vi "Main.vi"() -> ()   [LabVIEW 2019]
uses:
  Controls/State.ctl
  <vilib>/MediaMongrels Ltd/WebSockets/WebSockets/WebSocket Server/WebSocket Server.lvclass
  <vilib>/MediaMongrels Ltd/WebSockets/Sockets/VISA TCP Listener/VISA TCP Listener.lvclass
panel:
  in  "Stop":bool
  out "Current Time":string
  # "Raspberry Pi WebSocket Server Example"
  # "This simple example sends the current date/time to the connected WebSocket Client.\n\nTo be used in conjunction with the corresponding NXG WebVI."
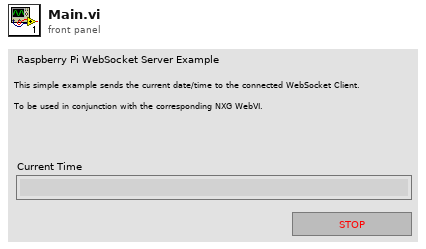
[diagram p1: front panel]
types:
  T1 = typedef "State.ctl" = enum16{"Initialise", "Listen", "Write Data", "Close WebSocket", "Exit"}
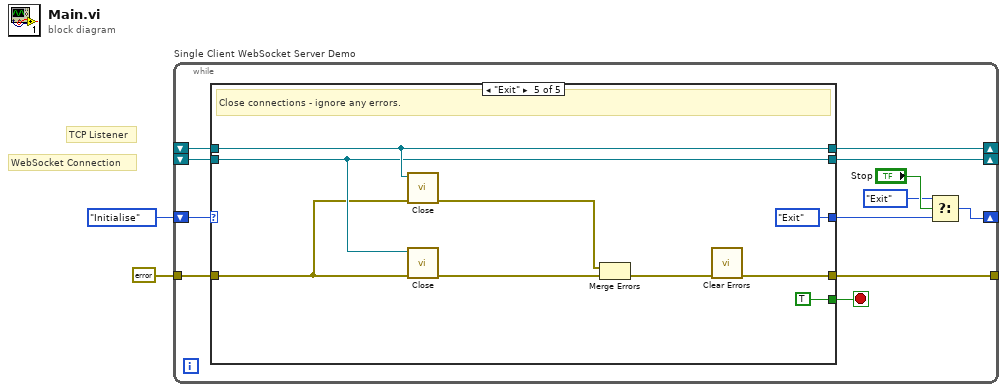
[diagram p0: block diagram]
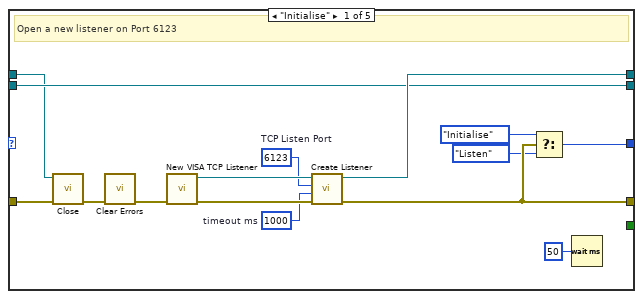
[diagram p2: hidden frame]
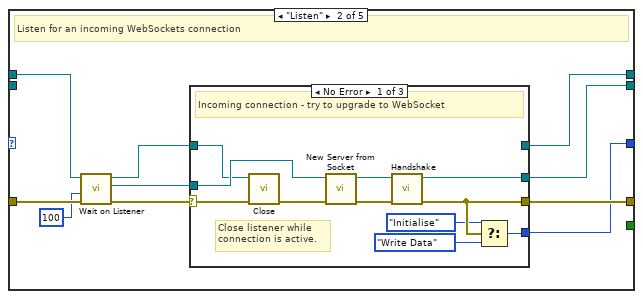
[diagram p3: hidden frame]
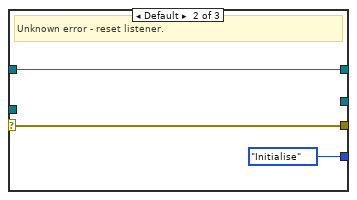
[diagram p4: hidden frame]
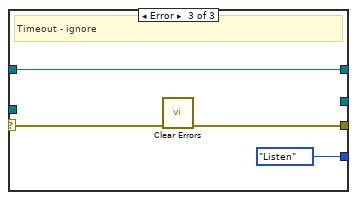
[diagram p5: hidden frame]
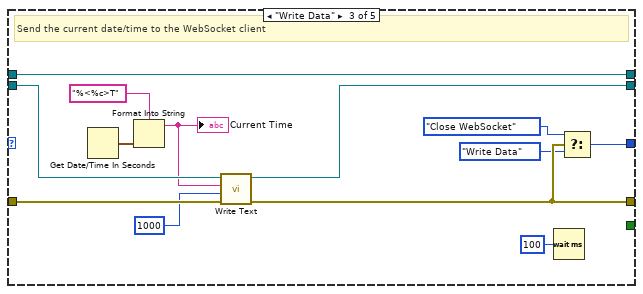
[diagram p6: hidden frame]
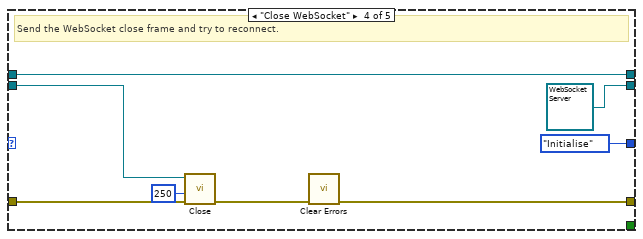
[diagram p7: hidden frame]
diagram:
  # "WebSocket Connection"
  # "TCP Listener"
  n1 = while "Single Client WebSocket Server Demo" {
    shift-right: [w13] -> _
    shift-left: _ -> [w10]
    tunnel: errorcluster {"status"=FALSE, "code"=0, "source"=""} ("error constant") -> [w11]
    tunnel: [w12] -> _
    shift-right: [w3] -> _
    shift-left: State."Initialise" -> [w14]
    shift-right: [w9] -> _
    shift-left: _ -> [w8]
    stop <- w7 stop-if-true
    n2 = case shown="\"Exit\"" w14 {
      tunnel: [w26 w31 w70 w78 w87] -> w13
      tunnel: [w24 w33 w61 w72 w79] -> w12
      tunnel: w11 -> [w18 w36 w69 w77 w80]
      tunnel: [w22 w30 w62 State."Initialise" State."Exit"] -> w4
      tunnel: w10 -> [w17 w35 w70 w78 w87]
      tunnel: [w19 w34 w66 refnum<class "WebSocket Server.lvclass"> refnum ("WebSocket out") w83] -> w9
      tunnel: w8 -> [w19 _ w68 w76 w83]
      tunnel: [_ _ _ _ TRUE] -> w7
      frame "Initialise" {
        w21 = 1000  # timeout ms
        w27 = u16 6123  # TCP Listen Port
        # "Open a new listener on Port 6123"
        n3 = call-dynamic "Close.vi"("error in (no error)"=w18, "VISA TCP Listener in"=w17) -> ("error out"=w16:errorcluster)  [unwired: 9 in]
        n4 = call <vilib>:"Clear Errors.vi"("error in (no error)"=w16) -> ("error out"=w15:errorcluster)  [unwired: 5 in, 1 out]
        n5 = call <vilib>:"New VISA TCP Listener.vi"("error in (no error)"=w15) -> ("error out"=w28:errorcluster, "VISA TCP Listener out"=w29:refnum<class "VISA TCP Listener.lvclass">)  [unwired: 9 in]
        n6 = call-dynamic "Create Listener.vi"("error in (no error)"=w28, "timeout ms (5000)"=w21, "Port"=w27, "VISA TCP Listener in"=w29) -> ("error out"=w24:errorcluster, "VISA TCP Listener out"=w26:refnum<class "VISA TCP Listener.lvclass">)  [unwired: 6 in]
        n7 = Select(t=State."Initialise", s=w24, f=State."Listen") -> (s? t:f=w22:T1)
        n8 = Wait (ms)(milliseconds to wait=u32 50) -> ()  [unwired: 1 out]
      }
      frame "Listen" {
        # "Listen for an incoming WebSockets connection"
        n9 = call-dynamic "Wait on Listener.vi"("error in (no error)"=w36, "timeout ms (5000)"=100, "VISA TCP Listener in"=w35) -> ("error out"=w38:errorcluster, "Socket out"=w39:refnum<class "Socket.lvclass">, "VISA TCP Listener out"=w37:refnum<class "VISA TCP Listener.lvclass">)  [unwired: 6 in]
        n10 = case shown="No Error" w38 {
          selector: w38 -> [w46 w53 w57]
          tunnel: w39 -> [w48 _ _]
          tunnel: w37 -> [w45 w52 w56]
          tunnel: [w44 _ _] -> w34
          tunnel: [w43 w53 w54] -> w33
          tunnel: [_ w52 w56] -> w31
          tunnel: [w41 State."Initialise" State."Listen"] -> w30
          frame No Error {
            # "Close listener while connection is active."
            # "Incoming connection - try to upgrade to WebSocket"
            n11 = call-dynamic "Close.vi"("error in (no error)"=w46, "VISA TCP Listener in"=w45) -> ("error out"=w47:errorcluster)  [unwired: 9 in]
            n12 = call <vilib>:"New Server from Socket.vi"("error in (no error)"=w47, "Socket"=w48) -> ("error out"=w49:errorcluster, "WebSocket Server out"=w50:refnum<class "WebSocket Server.lvclass">)  [unwired: 8 in]
            n13 = call-dynamic "Handshake.vi"("error in (no error)"=w49, "WebSocket Connection in"=w50) -> ("error out"=w43:errorcluster, "WebSocket Connection out"=w44:refnum<class "WebSocket Server.lvclass">)  [unwired: 8 in]
            n14 = Select(t=State."Initialise", s=w43, f=State."Write Data") -> (s? t:f=w41:T1)
          }
          frame Default {
            # "Unknown error - reset listener."
          }
          frame Error {
            # "Timeout - ignore"
            n15 = call <vilib>:"Clear Errors.vi"("error in (no error)"=w57) -> ("error out"=w54:errorcluster)  [unwired: 5 in, 1 out]
          }
        }
      }
      frame "Write Data" {
        # "Send the current date/time to the WebSocket client"
        n16 = Get Date/Time In Seconds() -> (seconds since 1Jan1904=w65:timestamp)
        n17 = Format Into String(format string="%<%c>T", w65) -> (resulting string=w63:string)  [unwired: 2 in, 1 out]
        "Current Time" <- w63
        n18 = call-dynamic "Write Text.vi"("error in (no error)"=w69, "timeout ms (5000)"=1000, "String Data"=w63, "WebSocket in"=w68) -> ("error out"=w61:errorcluster, "WebSocket out"=w66:refnum<class "WebSocket Server.lvclass">)  [unwired: 6 in]
        n19 = Wait (ms)(milliseconds to wait=u32 100) -> ()  [unwired: 1 out]
        n20 = Select(t=State."Close WebSocket", s=w61, f=State."Write Data") -> (s? t:f=w62:T1)
      }
      frame "Close WebSocket" {
        # "Send the WebSocket close frame and try to reconnect."
        n21 = call-dynamic "Close.vi"("error in (no error)"=w77, "timeout ms (5000)"=250, "WebSocket in"=w76) -> ("error out"=w74:errorcluster)  [unwired: 8 in]
        n22 = call <vilib>:"Clear Errors.vi"("error in (no error)"=w74) -> ("error out"=w72:errorcluster)  [unwired: 5 in, 1 out]
      }
      frame "Exit" {
        # "Close connections - ignore any errors."
        n23 = call-dynamic "Close.vi"("error in (no error)"=w80, "VISA TCP Listener in"=w87) -> ("error out"=w85:errorcluster)  [unwired: 9 in]
        n24 = call-dynamic "Close.vi"("error in (no error)"=w80, "WebSocket in"=w83) -> ("error out"=w84:errorcluster)  [unwired: 9 in]
        n25 = Merge Errors(w85, w84) -> (w86:errorcluster)
        n26 = call <vilib>:"Clear Errors.vi"("error in (no error)"=w86) -> ("error out"=w79:errorcluster)  [unwired: 5 in, 1 out]
      }
    }
    n27 = Select(t=State."Exit", s="Stop", f=w4) -> (s? t:f=w3:T1)
  }
